vi "CH375_Test.vi"() -> ()   [LabVIEW 2020]
uses:
  Global_CH375.vi
panel:
  in  "退出":bool
  in  "移动速度":u16(ring)=1 items=["1", "1/2", "1/4", "1/8", "1/16", "1/32", "1/64", "1/128"]
  out "设备状态":bool
  out "当前角度":dbl
  in  "相对位置":dbl
  in  "绝对位置":dbl
  in  "设置相对位置":bool
  in  "设置绝对位置":bool
  in  "重置当前角度":bool
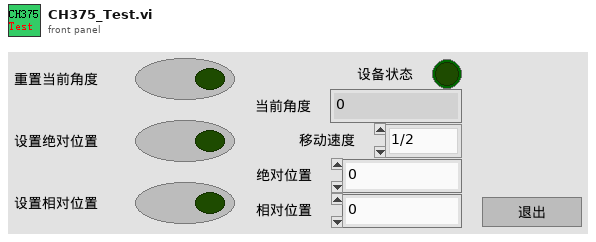
[diagram p1: front panel]
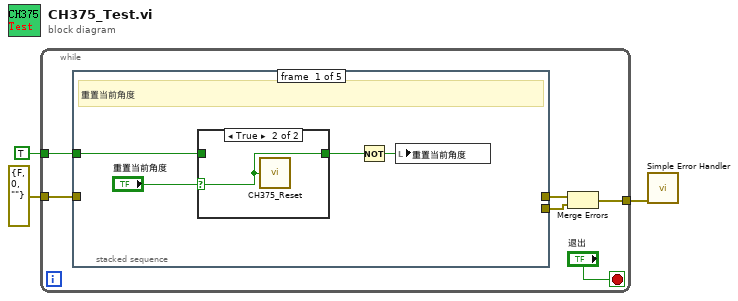
[diagram p0: block diagram]
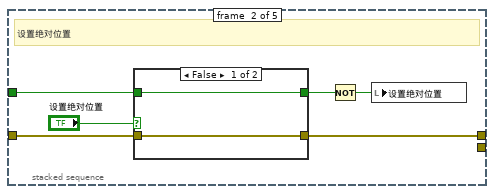
[diagram p3: hidden frame]
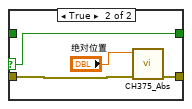
[diagram p4: hidden frame]
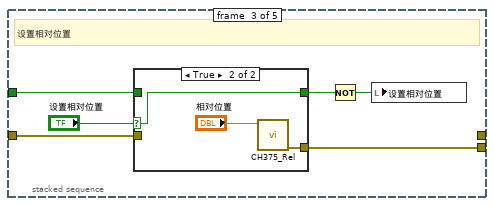
[diagram p5: hidden frame]
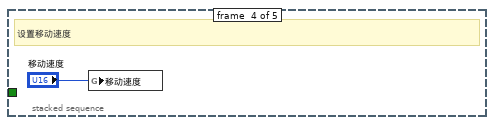
[diagram p7: hidden frame]
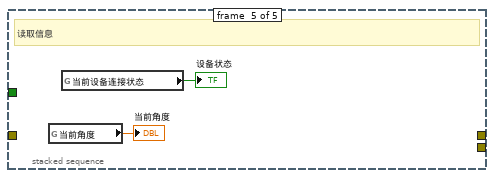
[diagram p8: hidden frame]
diagram:
  n1 = while {
    tunnel: errorcluster {"status"=FALSE, "code"=0, "source"=""} ("error constant") -> [w9]
    tunnel: [w8] -> w3
    tunnel: TRUE -> [w5]
    stop <- "退出" stop-if-true
    n2 = stacked-sequence {
      tunnel: w9 -> [_ w17 w29 _ _]
      tunnel: [_ w18 _ _ _] -> w7
      tunnel: [_ _ w30 _ _] -> w6
      tunnel: w5 -> [w10 w16 w28 _ _]
      frame #0 {
        # "重置当前角度"
        n3 = case shown="True" "重置当前角度" {
          selector: "重置当前角度" -> [_ w15]
          tunnel: [w14 w15] -> w12
          tunnel: w10 -> [w14 _]
          frame False {
          }
          frame True {
            n4 = call "CH375_Reset.vi"("Reset"=w15) -> ()
          }
        }
        n5 = Not(x=w12) -> (.not. x?=w13:bool)
        n6 = local write "重置当前角度"(w13) -> ()
      }
      frame #1 {
        # "设置绝对位置"
        n7 = case shown="False" "设置绝对位置" {
          selector: "设置绝对位置" -> [_ w27]
          tunnel: [w22 w27] -> w20
          tunnel: w17 -> [w23 w26]
          tunnel: [w23 w24] -> w18
          tunnel: w16 -> [w22 _]
          frame False {
          }
          frame True {
            n8 = call "CH375_Abs.vi"("Error In"=w26, "旋转角度"="绝对位置") -> ("Error Out"=w24:errorcluster)  [unwired: 9 in]
          }
        }
        n9 = Not(x=w20) -> (.not. x?=w19:bool)
        n10 = local write "设置绝对位置"(w19) -> ()
      }
      frame #2 {
        # "设置相对位置"
        n11 = case shown="True" "设置相对位置" {
          selector: "设置相对位置" -> [_ w38]
          tunnel: [w34 w38] -> w33
          tunnel: [w35 w37] -> w30
          tunnel: w29 -> [w35 _]
          tunnel: w28 -> [w34 _]
          frame False {
          }
          frame True {
            n12 = call "CH375_Rel.vi"("移动步长"="相对位置") -> ("Error Out"=w37:errorcluster)  [unwired: 10 in]
          }
        }
        n13 = Not(x=w33) -> (.not. x?=w31:bool)
        n14 = local write "设置相对位置"(w31) -> ()
      }
      frame #3 {
        # "设置移动速度"
        n15 = global write "Global_CH375.vi" "移动速度"("移动速度") -> ()
      }
      frame #4 {
        # "读取信息"
        n16 = global read "Global_CH375.vi" "当前角度"() -> (→"当前角度":dbl)
        n17 = global read "Global_CH375.vi" "当前设备连接状态"() -> (→"设备状态":bool)
      }
    }
    n18 = Merge Errors(w7, w6) -> (w8:errorcluster)
  }
  n19 = call <vilib>:"Simple Error Handler.vi"("error in (no error)"=w3) -> ()  [unwired: 4 in, 5 out]
